vi "acquire multi waves by LAN init subvi.vi"(8 "error in (no error)":errorcluster, 11 "TCP Network Connection in":refnum<k5>) -> (0 "error out":errorcluster, 1 "SEC/DIV":string, 2 "data out 2":string, 3 "TCP Network Connection out":refnum<k5>, 4 "CH1":string, 5 "data out":string)   [LabVIEW 2013]
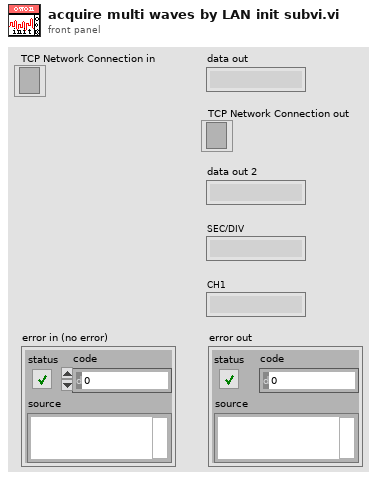
[diagram p1: front panel]
types:
  T1 = enum16{"Standard", "Buffered", "CRLF", "Immediate"}
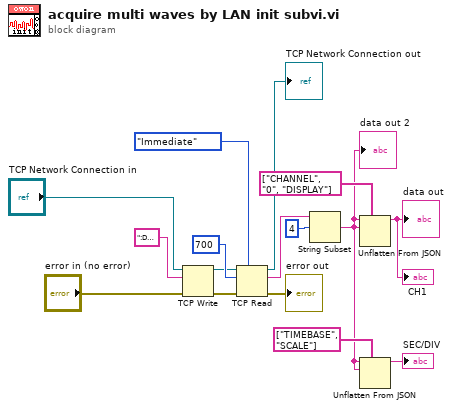
[diagram p0: block diagram]
diagram:
  n1 = TCP Write(connection ID="TCP Network Connection in", data in=":DATA:WAVE:SCREEN:HEAD?" ("ID Query"), error in (no error)="error in (no error)") -> (connection ID out=w7:refnum<k5>, error out=w8:errorcluster)  [unwired: 1 in, 1 out]
  n2 = TCP Read(connection ID=w7, bytes to read=u32 700 ("byte count"), error in (no error)=w8, 7:T1."Immediate" ("mode (standard)")) -> (connection ID out=→"TCP Network Connection out":refnum<k5>, data out=w14:string, error out=→"error out":errorcluster)  [unwired: 1 in]
  n3 = String Subset(string=w14, offset (0)=4) -> (substring=w1:string)  [unwired: 1 in]
  "data out 2" <- w1
  n4 = Unflatten From JSON(path=string[] ["CHANNEL", "0", "DISPLAY"], JSON string=w1, type and defaults=w1) -> (value=→"CH1" →"data out":string)  [unwired: 4 in, 1 out]
  n5 = Unflatten From JSON(path=string[] ["TIMEBASE", "SCALE"], JSON string=w1, type and defaults=w1) -> (value=→"SEC/DIV":string)  [unwired: 4 in, 1 out]
